vi "Query_TCPinfo.vi"(11 "AccelNET.lvlib:TCP.lvclass":refnum<class "TCP.lvclass">) -> (0 "timeout ms (60000)":i32, 1 "Write Port":i16, 2 "Read Port":i16, 3 "IP Address":string, 4 "Write ID":refnum<k5>, 5 "Read ID":refnum<k5>)   [LabVIEW 2012, in "AccelNET.lvlib" / "TCP.lvclass"]
uses:
  TCP.lvclass
  TCP.lvclass/TCP.ctl
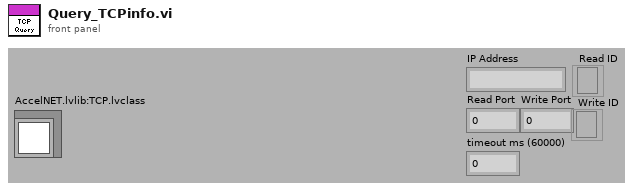
[diagram p1: front panel]
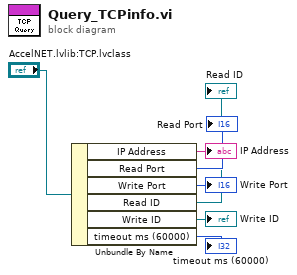
[diagram p0: block diagram]
diagram:
  n1 = Unbundle By Name("AccelNET.lvlib:TCP.lvclass") -> ("IP Address"=→"IP Address":string, "Read Port"=→"Read Port":i16, "Write Port"=→"Write Port":i16, "Read ID"=→"Read ID":refnum<k5>, "Write ID"=→"Write ID":refnum<k5>, "timeout ms (60000)"=→"timeout ms (60000)":i32)
